vi "niScope EX Getting Started.vi"() -> ()   [LabVIEW 2021]
doc: "Example: Getting Started\n\nRecommended Input Signal: 100 kHz, 1.8 Vpp, sine wave\n\nDevices Supported: Refer to NI Example Finder\n\nLabVIEW Description:\n\nThis example opens a session to the NI-SCOPE driver by passing in the device's resource name to the Initialize VI. The resource name is a unique identifier for your National Instruments' hardware product. It can be found (and changed) by running Measurement & Automation Explorer (MAX). A shortcut to MAX is placed on your desktop when NI-SCOPE or NI-DAQ is installed.\n\nThe session handle returned from the Initialize VI is a parameter to all VIs in the NI-SCOPE driver. Only one session may be opened at a time for your oscilloscope, and every session should be closed by calling the Close vi. The session should be closed even when an error occurs.\n\nThe Auto Setup VI takes several acquisitions to measure the amplitude and frequency of the input signal. This allows it to optimally set properties such as the sample rate, vertical range, and minimum record length. The Read VI, initiates an acquisition, waits for it to finish, and fetches the data from the oscilloscope. The data is returned as a bundle of the initial x, x increment, and waveform. Initial x is the time of the first point in the waveform relative to the trigger, while the x increment is the time between two points in the waveform. This bundle may be directly wired to a waveform graph, to display the waveform with timing information. \n\nThe Error Handler VI translates any error messages into text messages."
uses:
  <instrlib>/niScope/Acquire/niScope Multi Read Cluster.vi
  <instrlib>/niDigital/niDigital.llb/niDigital Selected Function.ctl
  <instrlib>/niDigital/niDigital.llb/niDigital Get Site Results Site Numbers.vi
  <instrlib>/niDigital/niDigital.llb/niDigital Burst Pattern (Pass Fail).vi
panel:
  in  "Scope Channel(s) 2":string="0" caption="Scope Channel(s)"
  in  "Scope 2":refnum<k15>="Dev1" caption="Resource Name(s)"
  out "Waveform Graph 2":T1(graph) caption="Waveform Graph"
  in  "Digital 2":refnum<k15>="PXI1Slot2,PXI1Slot3" caption="resource name"
  out "Pass? 2":bool[](array[boolean])
  out "Site 2":string[](array[string])
  in  "error in":errorcluster
  out "error out":errorcluster
  out "Site":string[](array[string])
  out "Pass?":bool[](array[boolean])
  in  "Digital":refnum<k15>="PXI1Slot2,PXI1Slot3" caption="resource name"
  out "Waveform Graph":T1(graph)
  in  "Scope":refnum<k15>="Dev1" caption="Resource Name(s)"
  in  "Scope Channel(s)":string="0"
  # "Overview: Demonstrates the minimal code needed to use NI-SCOPE.\nRequirements: NI-SCOPE\nInstructions: \n1.  Select the appropriate device in the Resource Name control.\n2.  Enter the channels you would like to acquire from in the Channel(s) control.\n3.  Run the VI."
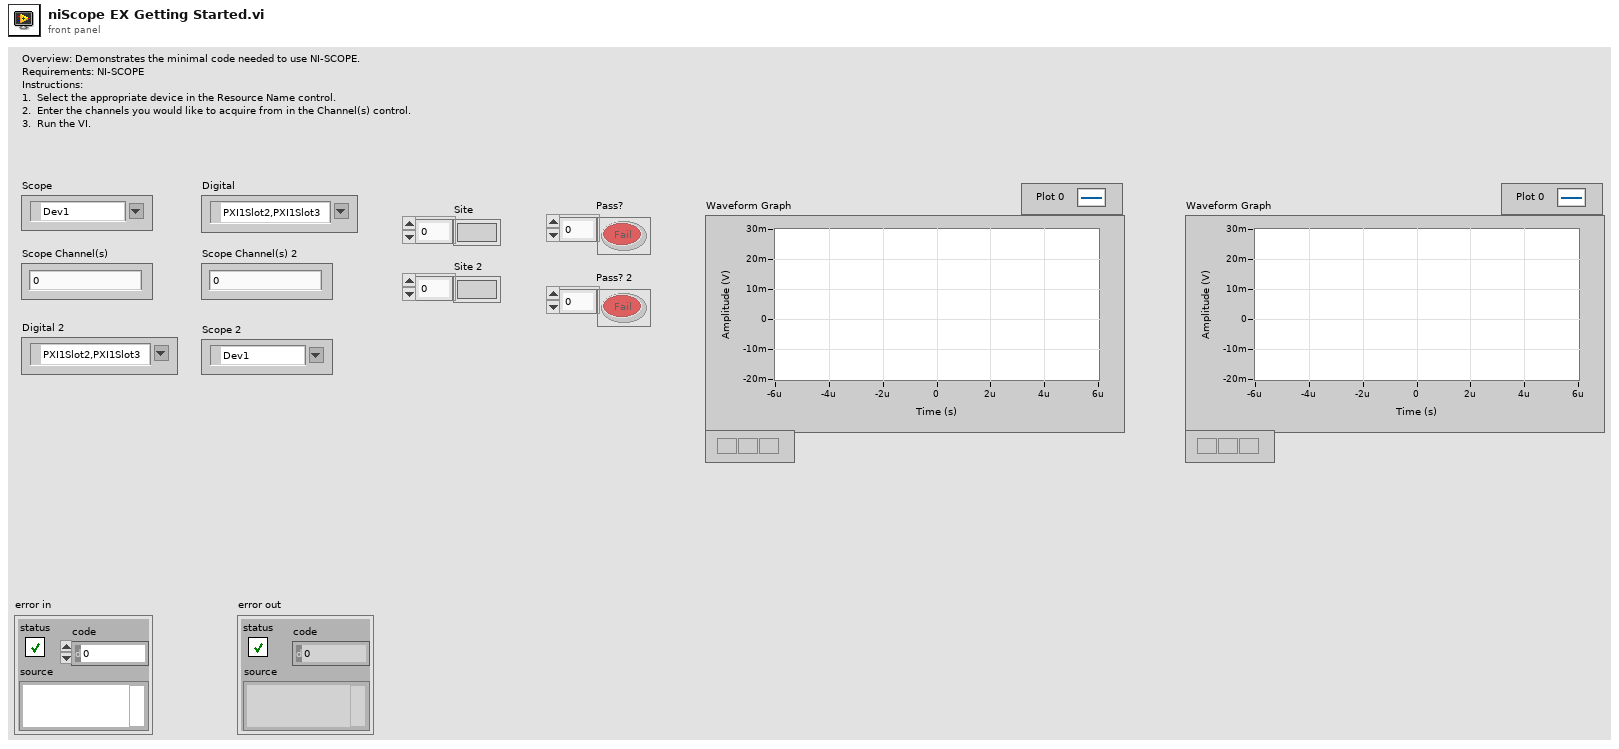
[diagram p1: front panel]
types:
  T1 = cluster{"relativeInitialX":dbl, "xIncrement":dbl, "wfm":dbl[]}[]
  T2 = typedef "niDigital Selected Function.ctl" = i32
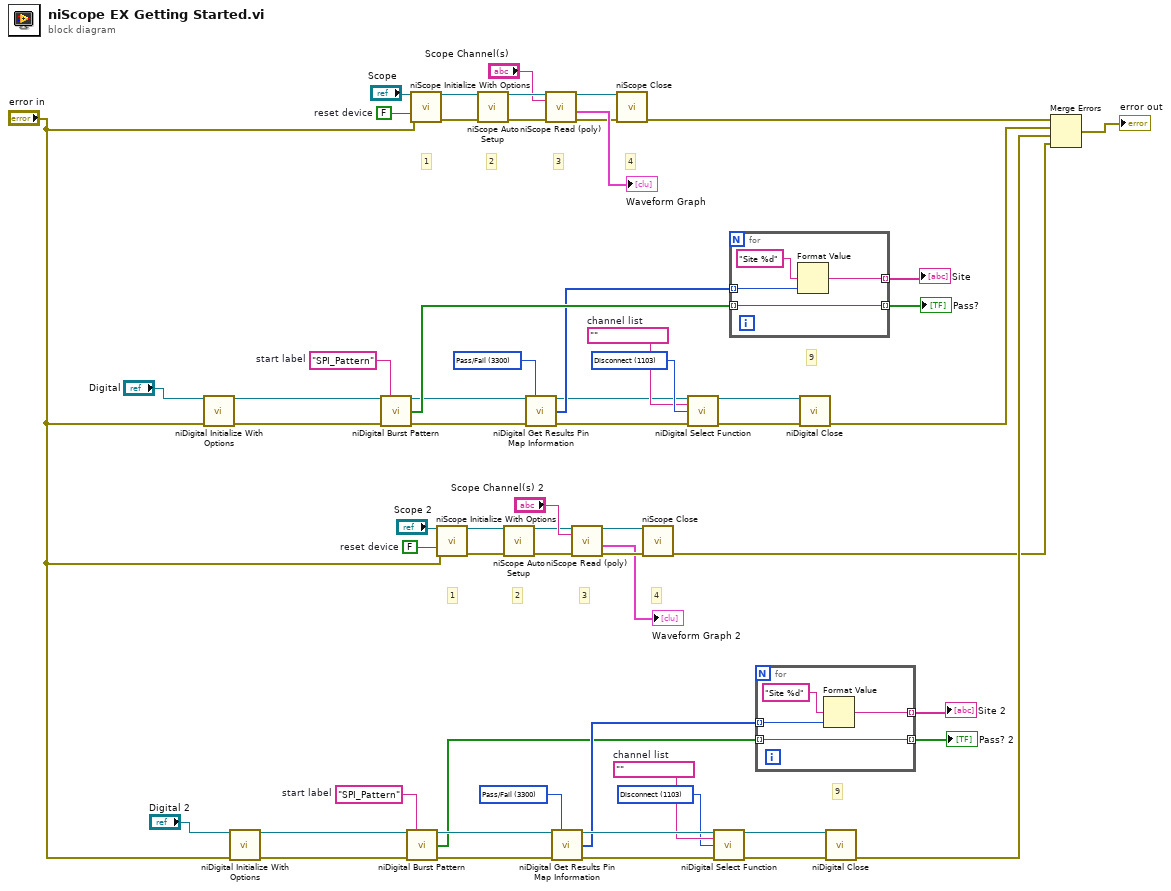
[diagram p0: block diagram]
diagram:
  w21 = ""  # channel list
  w20 = T2 1103 items=["Digital"=1100, "PPMU"=1101, "Off"=1102, "Disconnect"=1103] ("function")
  w15 = "SPI_Pattern"  # start label
  w19 = 3300 items=["Pass/Fail"=3300, "Capture Waveform"=3301] ("site result type")
  w7 = FALSE  # reset device
  w43 = ""  # channel list
  w44 = T2 1103 items=["Digital"=1100, "PPMU"=1101, "Off"=1102, "Disconnect"=1103] ("function")
  w49 = "SPI_Pattern"  # start label
  w45 = 3300 items=["Pass/Fail"=3300, "Capture Waveform"=3301] ("site result type")
  w57 = FALSE  # reset device
  # "9"
  # "4"
  # "3"
  # "2"
  # "1"
  # "9"
  # "4"
  # "3"
  # "2"
  # "1"
  n1 = call <instrlib>:"niDigital Initialize With Options.vi"("resource name"="Digital", "error in"="error in") -> ("instrument handle"=w37:refnum<k15>, "error out"=w36:errorcluster)  [unwired: 12 in]
  n2 = call <instrlib>:"niDigital Initialize With Options.vi"("resource name"="Digital 2", "error in"="error in") -> ("instrument handle"=w27:refnum<k15>, "error out"=w28:errorcluster)  [unwired: 12 in]
  n3 = call-poly <instrlib>:"niDigital Burst Pattern.vi"("instrument handle"=w37, "start label"=w49, "error in"=w36) -> ("instrument handle out"=w48:refnum<k15>, "pass"=w50:bool[], "error out"=w47:errorcluster)  [unwired: 10 in]
  n4 = call-poly <instrlib>:"niDigital Burst Pattern.vi"("instrument handle"=w27, "start label"=w15, "error in"=w28) -> ("instrument handle out"=w16:refnum<k15>, "pass"=w14:bool[], "error out"=w17:errorcluster)  [unwired: 10 in]
  n5 = call <instrlib>:"niScope Initialize With Options.vi"("resource name"="Scope", "reset device"=w57, "error in"="error in") -> ("instrument handle"=w60:refnum<k15>, "error out"=w59:errorcluster)  [unwired: 11 in]
  n6 = call <instrlib>:"niScope Initialize With Options.vi"("resource name"="Scope 2", "reset device"=w7, "error in"="error in") -> ("instrument handle"=w4:refnum<k15>, "error out"=w5:errorcluster)  [unwired: 11 in]
  n7 = call <instrlib>:"niScope Auto Setup.vi"("instrument handle"=w60, "error in"=w59) -> ("instrument handle out"=w56:refnum<k15>, "error out"=w55:errorcluster)  [unwired: 12 in]
  n8 = call <instrlib>:"niScope Auto Setup.vi"("instrument handle"=w4, "error in"=w5) -> ("instrument handle out"=w8:refnum<k15>, "error out"=w9:errorcluster)  [unwired: 12 in]
  n9 = call-poly <instrlib>:"niDigital Get Results Pin Map Information.vi"("instrument handle"=w48, "site result type"=w45, "error in"=w47) -> ("instrument handle out"=w42:refnum<k15>, "site numbers"=w46:i32[], "error out"=w41:errorcluster)  [unwired: 10 in]
  n10 = call-poly <instrlib>:"niScope Read (poly).vi"("error in"=w55, "channels"="Scope Channel(s)", "instrument handle"=w56) -> ("error out"=w52:errorcluster, "waveform"=→"Waveform Graph":T1, "instrument handle out"=w51:refnum<k15>)  [unwired: 5 in, 1 out]
  n11 = call-poly <instrlib>:"niDigital Get Results Pin Map Information.vi"("instrument handle"=w16, "site result type"=w19, "error in"=w17) -> ("instrument handle out"=w22:refnum<k15>, "site numbers"=w18:i32[], "error out"=w23:errorcluster)  [unwired: 10 in]
  n12 = call-poly <instrlib>:"niScope Read (poly).vi"("error in"=w9, "channels"="Scope Channel(s) 2", "instrument handle"=w8) -> ("error out"=w12:errorcluster, "waveform"=→"Waveform Graph 2":T1, "instrument handle out"=w13:refnum<k15>)  [unwired: 5 in, 1 out]
  n13 = call <instrlib>:"niScope Close.vi"("instrument handle"=w51, "error in"=w52) -> ("error out"=w33:errorcluster)  [unwired: 13 in]
  n14 = call <instrlib>:"niScope Close.vi"("instrument handle"=w13, "error in"=w12) -> ("error out"=w1:errorcluster)  [unwired: 13 in]
  n15 = call <instrlib>:"niDigital Select Function.vi"("instrument handle"=w42, "channel list"=w43, "function"=w44, "error in"=w41) -> ("instrument handle out"=w39:refnum<k15>, "error out"=w40:errorcluster)  [unwired: 10 in]
  n16 = call <instrlib>:"niDigital Select Function.vi"("instrument handle"=w22, "channel list"=w21, "function"=w20, "error in"=w23) -> ("instrument handle out"=w25:refnum<k15>, "error out"=w24:errorcluster)  [unwired: 10 in]
  n17 = for {
    tunnel: w50 -> [w61] mode=indexing
    tunnel: w46 -> [w63] mode=indexing
    tunnel: [w62] -> w35 mode=indexing
    tunnel: [w61] -> w34 mode=indexing
    n18 = Format Value(format string="Site %d", value (0)=w63) -> (output string=w62:string)  [unwired: 1 in]
  }
  "Pass?" <- w34
  "Site" <- w35
  n19 = for {
    tunnel: w14 -> [w65] mode=indexing
    tunnel: w18 -> [w67] mode=indexing
    tunnel: [w66] -> w29 mode=indexing
    tunnel: [w65] -> w30 mode=indexing
    n20 = Format Value(format string="Site %d", value (0)=w67) -> (output string=w66:string)  [unwired: 1 in]
  }
  "Pass? 2" <- w30
  "Site 2" <- w29
  n21 = call <instrlib>:"niDigital Close.vi"("instrument handle"=w39, "error in"=w40) -> ("error out"=w31:errorcluster)  [unwired: 13 in]
  n22 = call <instrlib>:"niDigital Close.vi"("instrument handle"=w25, "error in"=w24) -> ("error out"=w2:errorcluster)  [unwired: 13 in]
  n23 = Merge Errors(w33, w31, w2, w1) -> (→"error out":errorcluster)
